vi "SL TAGS Add-Update Class Tag Properties.vi"(8 "error in (no error)":errorcluster, 11 "Tag In":T1={"Class Properties"={"Class Data Type"=enum."Double", "Name"="", "Description"="", "Interpolation Method"=enum."linear", "Unit of Measure"=enum."Hour", "Maximum Interpolation"="", "Role"=enum."Supervisor"}, "SL Tag"=refnum, "SystemLink Cluster"={"Path"="", "Data Type"=enum."Double", "Value"=variant, "Time Stamp"=timestamp(0 s since 1904-01-01)}, "Class Value"=variant}) -> (0 "error out":errorcluster, 3 "Tag Ref Out":T1={"Class Properties"={"Class Data Type"=enum."Double", "Name"="", "Description"="", "Interpolation Method"=enum."linear", "Unit of Measure"=enum."Hour", "Maximum Interpolation"="", "Role"=enum."Supervisor"}, "SL Tag"=refnum, "SystemLink Cluster"={"Path"="", "Data Type"=enum."Double", "Value"=variant, "Time Stamp"=timestamp(0 s since 1904-01-01)}, "Class Value"=variant})   [LabVIEW 2017, in "EEISysLink.lvclass"]
doc: "Add or update all the tag properties included in the SystemLink class data.\n\nJames Tillett P.E.\nEndeavor Engineering Inc.\nwww.endeavoreng.com"
uses:
  EEISysLink.lvclass
  Controls/SL Tag.ctl
  <vilib>/Skyline/Tag/Wrapper/Wrapper_class/NI Skyline Tag.lvclass
  Controls/SL Tag Properties.ctl
  Controls/SL Tag Data Type.ctl
  Controls/SL Tag Interpolation Method.ctl
  Controls/SL Tag Unit of Measure.ctl
  Controls/SL Tag Type.ctl
  <vilib>/Skyline/Tag/Shared/typedefs/Tag Cluster.ctl
  <vilib>/Skyline/Tag/Shared/typedefs/DataType.ctl
  <vilib>/Skyline/Tag/Shared/typedefs/TagProperty.ctl
  <vilib>/Skyline/Tag/Shared/NI Skyline Tag.lvlib
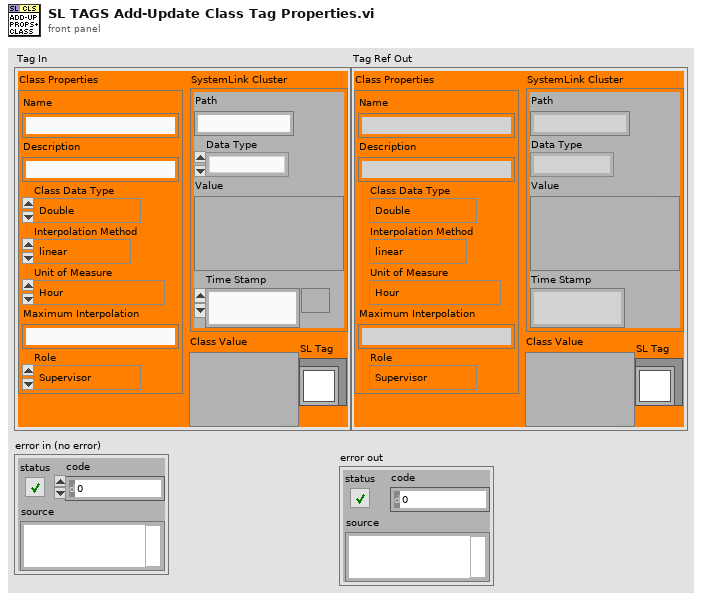
[diagram p1: front panel]
types:
  T1 = typedef "EEISysLink.lvclass/SL Tag.ctl" = cluster{"Class Properties":T2, "SL Tag":refnum<class "NI Skyline Tag.lvclass">, "SystemLink Cluster":T7, "Class Value":variant}
  T2 = typedef "EEISysLink.lvclass/SL Tag Properties.ctl" = cluster{"Class Data Type":T3, "Name":string, "Description":string, "Interpolation Method":T4, "Unit of Measure":T5, "Maximum Interpolation":string, "Role":T6}
  T3 = typedef "EEISysLink.lvclass/SL Tag Data Type.ctl" = enum16{"Double", "Integer", "String", "Boolean", "Waveform"}
  T4 = typedef "EEISysLink.lvclass/SL Tag Interpolation Method.ctl" = enum16{"linear", "pilinear", "step"}
  T5 = typedef "EEISysLink.lvclass/SL Tag Unit of Measure.ctl" = enum16{"no units", "Second", "Hour", "Minute", "Day", "Year", "Month", "Week", "Foot", "Yard", "Meter", "Centimeter", "Inch", "Mile", "Nautical Mile", "Miles per Hour", "Meters per second", "Square meter", "Cubic meter", "Cubic centimeter", "Cubic inch", "Liter", "Gallon", "Gallons dry US", "Gallon UK", "Percent", "Revolutions per minute", "Revolution", "Degree angle", "Astronomical Unit", "Atom", "Atomic mass", "Bar", "Byte", "C (speed of light)", "Curie", "Decibel", "Electron Volt", "Ounce", "Knot", "G", "Grade", "Are", "Hectare", "Faraday", "Franklin", "Gilbert", "Erg", "Lambert", "Maxwell", "Gauss", "Electron mass", "Kilogram force", "Pound force", "Rad", "Centiradian", "Sphere", "Mach", "Fluid Ounces", "Fluid Ounces UK", "Fahrenheit", "Celsius", "Kelvin", "Rankine", "Gram", "Kilogram", "Pound", "Short/US Ton", "Long/UK ton", "Metric ton", "Mole", "Pounds per square inch", "Inches water column", "Torr", "Millitorr", "Millimeter mercury", "Inches mercury", "Bar (2)", "Atmosphere", "Pascal", "Watt", "kiloWatt", "Horsepower", "Kilowatt Hour", "British thermal units", "Millions of BTU", "Ampere", "Candela", "Radian", "Steradian", "Bit", "Hertz", "Newton", "Joule", "Coulomb", "Volt", "Farad", "Ohm", "Siemens", "Weber", "Tesla", "Henry", "Lumen", "Lux", "Becqueral", "Gray", "Sievert", "Katal", "Angstrom", "Light Year", "Parsec", "Point", "Pixel", "Dyne", "Kilogram force (2)", "Pound force (2)", "Rem", "Rutherford", "Roentgen"}
  T6 = typedef "EEISysLink.lvclass/SL Tag Type.ctl" = enum16{"All", "Supervisor", "Worker"}
  T7 = typedef "NI Skyline Tag.lvlib/Tag Cluster.ctl" = cluster{"Path":string, "Data Type":T8, "Value":variant, "Time Stamp":timestamp}
  T8 = typedef "NI Skyline Tag.lvlib/DataType.ctl" = enum32{"Double", "Integer", "String"}
  T9 = typedef "NI Skyline Tag.lvlib/TagProperty.ctl" = cluster{"key":string, "value":string}
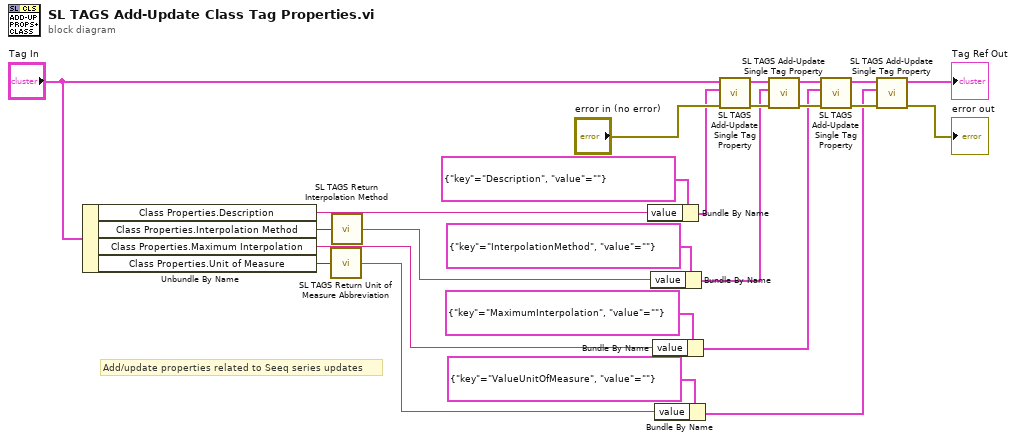
[diagram p0: block diagram]
diagram:
  # "Add/update properties related to Seeq series updates"
  n1 = Unbundle By Name("Tag In") -> ("Class Properties.Description"=w22:string, "Class Properties.Interpolation Method"=w24:T4, "Class Properties.Maximum Interpolation"=w20:string, "Class Properties.Unit of Measure"=w23:T5)
  n2 = call "SL TAGS Return Unit of Measure Abbreviation.vi"("Unit of Measure"=w23) -> ("Seeq Unit of Measure Abbreviation"=w19:string)  [unwired: 4 in]
  n3 = call "SL TAGS Return Interpolation Method.vi"("Interpolation Method"=w24) -> ("Seeq Interpolation Method"=w21:string)  [unwired: 4 in]
  n4 = Bundle By Name(cluster=T9 {"key"="Description", "value"=""} ("Tag Property In"), "value"=w22) -> (w17:T9)
  n5 = Bundle By Name(cluster=T9 {"key"="InterpolationMethod", "value"=""} ("Tag Property In"), "value"=w21) -> (w10:T9)
  n6 = Bundle By Name(cluster=T9 {"key"="MaximumInterpolation", "value"=""} ("Tag Property In"), "value"=w20) -> (w9:T9)
  n7 = Bundle By Name(cluster=T9 {"key"="ValueUnitOfMeasure", "value"=""} ("Tag Property In"), "value"=w19) -> (w8:T9)
  n8 = call "SL TAGS Add-Update Single Tag Property.vi"("error in (no error)"="error in (no error)", "Tag Property In"=w17, "Tag Ref In"="Tag In") -> ("error out"=w15:errorcluster, "Tag Ref Out"=w16:T1)  [unwired: 6 in, 1 out]
  n9 = call "SL TAGS Add-Update Single Tag Property.vi"("error in (no error)"=w15, "Tag Property In"=w10, "Tag Ref In"=w16) -> ("error out"=w13:errorcluster, "Tag Ref Out"=w14:T1)  [unwired: 6 in, 1 out]
  n10 = call "SL TAGS Add-Update Single Tag Property.vi"("error in (no error)"=w13, "Tag Property In"=w9, "Tag Ref In"=w14) -> ("error out"=w11:errorcluster, "Tag Ref Out"=w12:T1)  [unwired: 6 in, 1 out]
  n11 = call "SL TAGS Add-Update Single Tag Property.vi"("error in (no error)"=w11, "Tag Property In"=w8, "Tag Ref In"=w12) -> ("error out"=→"error out":errorcluster, "Tag Ref Out"=→"Tag Ref Out":T1)  [unwired: 6 in, 1 out]
